vi "Launch.vi"(7 "Open FP":bool=TRUE, 8 "error in (no error)":errorcluster, 9 "Name":string, 10 "vi path":path, 11 "Controller in":refnum<class "Controller.lvclass">) -> (0 "error out":errorcluster, 3 "Controller out":refnum<class "Controller.lvclass">)   [LabVIEW 2020, in "Controller.lvclass"]
uses:
  Controller.lvclass
  Controller.lvclass/Controller.ctl
  Module/Module.lvclass/Module.ctl
  Module/Get Name.vi
  <vilib>/ErrorRing/Error Ring.xnode
  Module/Module.lvclass
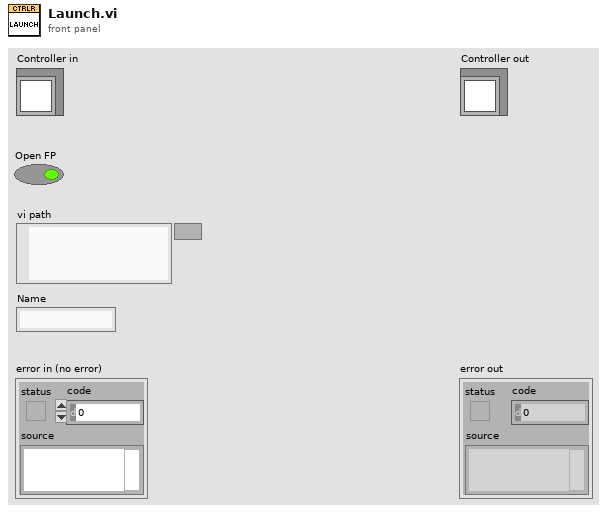
[diagram p1: front panel]
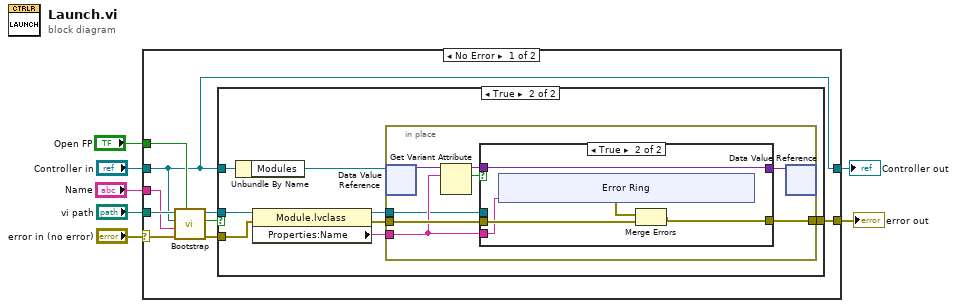
[diagram p0: block diagram]
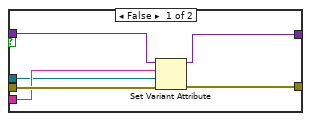
[diagram p3: hidden frame]
diagram:
  n1 = case shown="No Error" "error in (no error)" {
    selector: "error in (no error)" -> [w13 w51]
    tunnel: [w15 w51] -> w6
    tunnel: [w9 w50] -> w4
    tunnel: "Controller in" -> [w9 w50]
    tunnel: "vi path" -> [w14 _]
    tunnel: "Open FP" -> [w12 _]
    tunnel: "Name" -> [w8 _]
    frame No Error {
      n2 = call "Bootstrap.vi"("Open FP"=w12, "error in (no error)"=w13, "Name"=w8, "Controller.lvclass"=w9, "vi path"=w14) -> ("error out"=w11:errorcluster, "Is Running?"=w10:bool, "Module out"=w16:refnum<class "Module.lvclass">)  [unwired: 4 in]
      n3 = case shown="True" w10 {
        tunnel: w9 -> [_ w25]
        tunnel: w11 -> [w17 w24]
        tunnel: w16 -> [_ w23]
        tunnel: [w17 w22] -> w15
        frame False {
        }
        frame True {
          n4 = Unbundle By Name(w25) -> ("Modules"=w21:refnum<data-value>)
          n5 = property class="Module.lvclass"(reference=w23, error in=w24) -> (reference out=w18:refnum<class "Module.lvclass">, error out=w19:errorcluster, "Properties:Name"=w20:string)
          n6 = in-place {
            in-place-border: w20 -> [w29]
            in-place-border: w19 -> [w32]
            in-place-border: w18 -> [w28]
            in-place-border: [w31] -> w22
            n7 = in-place-dvr #1(w21) -> (w30:variant)  [unwired: 1 out]
            n8 = Get Variant Attribute(Variant=w30, name=w29) -> (duplicate Variant=w27:variant, found=w26:bool)  [unwired: 2 in, 2 out]
            n9 = case shown="True" w26 {
              tunnel: [w39 w44] -> w33
              tunnel: w32 -> [w38 w42]
              tunnel: [w37 w43] -> w31
              tunnel: w29 -> [w36 w41]
              tunnel: w28 -> [w35 _]
              tunnel: w27 -> [w34 w44]
              frame False {
                n10 = Set Variant Attribute(Variant=w34, name=w36, value=w35, error in=w38) -> (Variant out=w39:variant, error out=w37:errorcluster)  [unwired: 1 out]
              }
              frame True {
                n11 = xnode "Error Ring"("parameter 0"=w41) -> ("error out"=w40:errorcluster)
                n12 = Merge Errors(w40, w42) -> (w43:errorcluster)
              }
            }
            n13 = in-place-dvr #1(w33) -> ()  [unwired: 2 out]
          }
        }
      }
    }
    frame Error {
    }
  }
  "error out" <- w6
  "Controller out" <- w4
